vi "to-string.vi"(8 "error in (no error)":errorcluster, 11 "UUID in":refnum<class "UUID.lvclass">) -> (0 "error out":errorcluster, 2 "uuid-string":string)   [LabVIEW 2020, in "graph.lvlib" / "UUID.lvclass"]
uses:
  UUID.lvclass
  UUID.lvclass/UUID.ctl
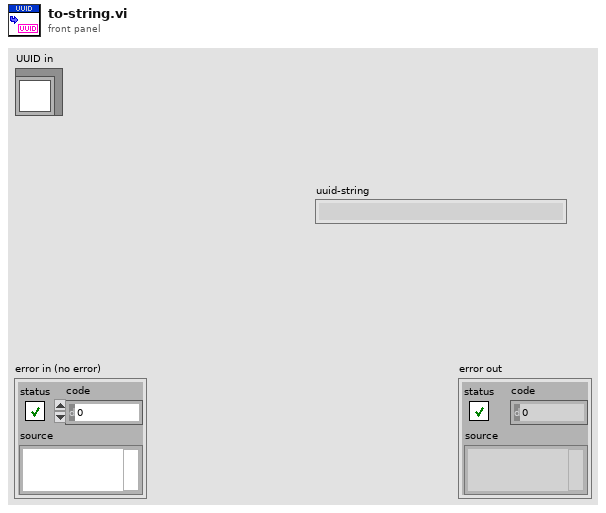
[diagram p1: front panel]
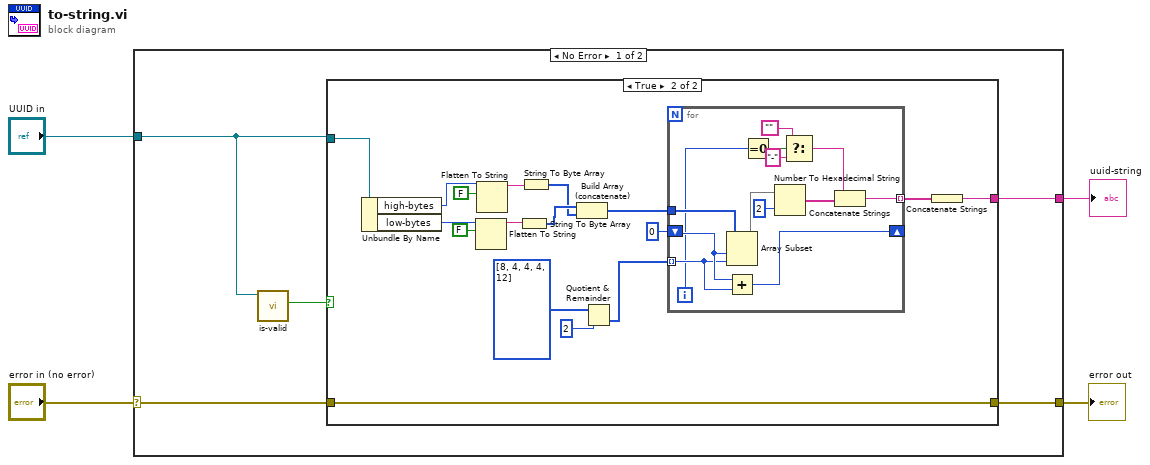
[diagram p0: block diagram]
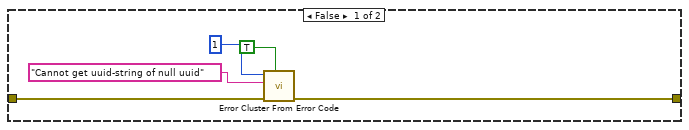
[diagram p2: hidden frame]
diagram:
  n1 = case shown="No Error" "error in (no error)" {
    selector: "error in (no error)" -> [w5 w45]
    tunnel: [w7 w45] -> w3
    tunnel: "UUID in" -> [w8 _]
    tunnel: [w9 _] -> w1
    frame No Error {
      n2 = call "is-valid.vi"("UUID in"=w8) -> ("is-valid?"=w6:bool)  [unwired: 10 in]
      n3 = case shown="True" w6 {
        tunnel: [_ w15] -> w9
        tunnel: w8 -> [_ w18]
        tunnel: [w12 w17] -> w7
        tunnel: w5 -> [w13 w17]
        frame False {
          n4 = call <vilib>:"Error Cluster From Error Code.vi"("show call chain? (False)"=TRUE, "error in (no error)"=w13, "error message (\"\")"="Cannot get uuid-string of null uuid" ("error message (\"\")"), "error code (0)"=1) -> ("error out"=w12:errorcluster)  [unwired: 5 in]
        }
        frame True {
          n5 = Unbundle By Name(w18) -> ("high-bytes"=w28:u64, "low-bytes"=w31:u64)
          n6 = Flatten To String(anything=w31, prepend array or string size? (T)=FALSE) -> (data string=w26:string)  [unwired: 2 in, 2 out]
          n7 = Flatten To String(anything=w28, prepend array or string size? (T)=FALSE) -> (data string=w27:string)  [unwired: 2 in, 2 out]
          n8 = String To Byte Array(string=w26) -> (unsigned byte array=w25:u8[])
          n9 = String To Byte Array(string=w27) -> (unsigned byte array=w24:u8[])
          n10 = Build Array (concatenate)(w25, w24) -> (w23:u8[])
          n11 = Quotient & Remainder(x=i32[] [8, 4, 4, 4, 12], y=2) -> (floor(x/y)=w19:i32[])  [unwired: 1 out]
          n12 = for {
            tunnel: w23 -> [w44]
            shift-right: [w41] -> _
            shift-left: 0 -> [w43]
            tunnel: w19 -> [w42] mode=indexing
            tunnel: [w32] -> w16 mode=indexing
            i -> [w40]
            n13 = Array Subset(array=w44, index=w43, length=w42) -> (w35:u8[])
            n14 = Add(x=w43, y=w42) -> (x+y=w41:i32)
            n15 = Equal To 0?(x=w40) -> (x = 0?=w39:bool)
            n16 = Number To Hexadecimal String(1:i16 2 ("width (-)"), 2:w35) -> (0:w34:string[])
            n17 = Select(t="", s=w39, f="-") -> (s? t:f=w36:string)
            n18 = Concatenate Strings(w36, w34) -> (w32:string)
          }
          n19 = Concatenate Strings(w16) -> (w15:string)
        }
      }
    }
    frame Error {
    }
  }
  "error out" <- w3
  "uuid-string" <- w1
